vi "Get Component Settings By ID.vi"(8 "error in (no error)":errorcluster, 10 "settings id":T1={"plugin"=-1, "thread"=-1, "group"=-1, "transfer"=-1, "channel"=-1}, 11 "Transfer Configuration in":refnum<class "Transfer Configuration.lvclass">) -> (0 "error out":errorcluster, 2 "component settings":T2[](array[typedef]), 3 "Transfer Configuration out":refnum<class "Transfer Configuration.lvclass">)   [LabVIEW 2019, in "DSF Core.lvlib" / "Transfer Configuration.lvclass"]
uses:
  Transfer Configuration.lvclass
  C:/Dev/GitHub/niveristand-data-sharing-framework-custom-device/Core/Classes/Configuration/Core/Core Configuration.lvclass
  Typedefs/DSF Settings Info.ctl
  Typedefs/DSF Configuration ID.ctl
  Transfer Configuration.lvclass/Transfer Configuration.ctl
  Core Configuration.lvclass
  DSF Core.lvlib
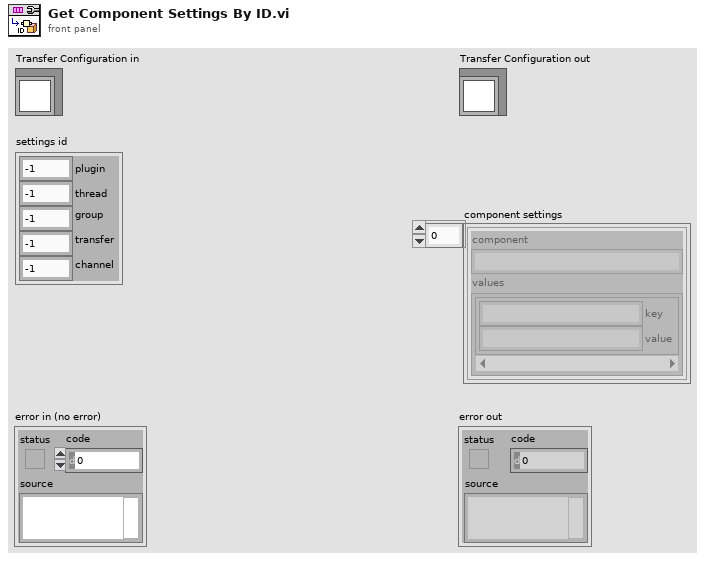
[diagram p1: front panel]
types:
  T1 = typedef "DSF Core.lvlib/DSF Configuration ID.ctl" = cluster{"plugin":i32, "thread":i32, "group":i32, "transfer":i32, "channel":i32}
  T2 = typedef "DSF Core.lvlib/DSF Settings Info.ctl" = cluster{"component":string, "values":cluster{"key":string, "value":string}[]}
  T3 = typedef "DSF Core.lvlib/Transfer Configuration.lvclass/Channel Configuration.ctl" = cluster{"configuration":T4, "component settings":T2[]}
  T4 = typedef "DSF Core.lvlib/Channel Configuration.lvclass/Core Channel Configuration.ctl" = cluster{"name":string, "units":string, "engine data type":T5, "string data type":T5, "string offset":u64}
  T5 = typedef "DSF Core.lvlib/DSF Data Type.ctl" = enum8{"Bool", "SGL", "DBL", "I8", "I16", "I32", "I64", "U8", "U16", "U32", "U64"}
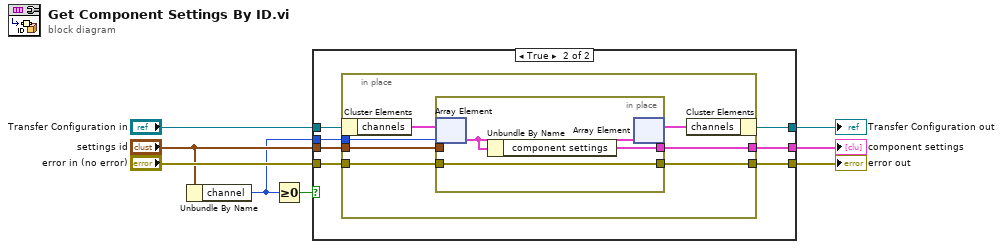
[diagram p0: block diagram]
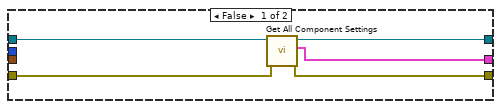
[diagram p2: hidden frame]
diagram:
  n1 = Unbundle By Name("settings id") -> ("channel"=w1:i32)
  n2 = Greater Or Equal To 0?(x=w1) -> (x >= 0?=w8:bool)
  n3 = case shown="True" w8 {
    tunnel: [w11 w14] -> w4
    tunnel: w1 -> [_ w16]
    tunnel: "error in (no error)" -> [w12 w20]
    tunnel: [w10 w19] -> w5
    tunnel: [w9 w18] -> w3
    tunnel: "settings id" -> [_ w17]
    tunnel: "Transfer Configuration in" -> [w13 w15]
    frame False {
      n4 = call "Get All Component Settings.vi"("error in (no error)"=w12, "Runtime Configuration in"=w13) -> ("error out"=w10:errorcluster, "component settings"=w9:T2[], "Runtime Configuration out"=w11:refnum<class "Transfer Configuration.lvclass">)  [unwired: 7 in]
    }
    frame True {
      n5 = in-place {
        in-place-border: w20 -> [w27]
        in-place-border: [w26] -> w19
        in-place-border: [w25] -> w18
        in-place-border: w17 -> [w24]
        in-place-border: w16 -> [w23]
        n6 = in-place-cluster #1(w15) -> ("channels"=w22:T3[])
        n7 = in-place {
          in-place-border: w27 -> [w30]
          in-place-border: [w30] -> w26
          in-place-border: [w29] -> w25
          in-place-border: w24 -> [_]
          n8 = in-place-array #2(w22, w23) -> (w28:T3)
          n9 = Unbundle By Name(w28) -> ("component settings"=w29:T2[])
          n10 = in-place-array #2(w28) -> (w21:T3[])  [unwired: 1 out]
        }
        n11 = in-place-cluster #1("channels"=w21) -> (w14:refnum<class "Transfer Configuration.lvclass">)
      }
    }
  }
  "error out" <- w5
  "Transfer Configuration out" <- w4
  "component settings" <- w3
